vi "Check AI Channel Settings.vi"(8 "error in":errorcluster, 9 "read channel settings":T1[](array[typedef]), 10 "initial channel settings":T1[](array[typedef]), 11 "TestCase in":refnum<class "TestCase.lvclass">) -> (0 "error out":errorcluster, 3 "TestCase out":refnum<class "TestCase.lvclass">)   [LabVIEW 2017, in "Module Test.lvclass"]
uses:
  Module Test Classes/Module Test.lvclass
  Scripting/Modules/Mode Classes/Controls/analog channel settings.ctl
  <vilib>/addons/_JKI Toolkits/VI Tester/TestCase.llb/TestCase.lvclass
  Scripting/Scan Engine Scripting.lvlib
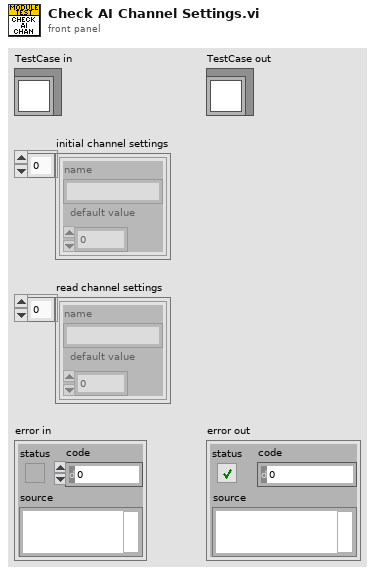
[diagram p1: front panel]
types:
  T1 = typedef "Scan Engine Scripting.lvlib/analog channel settings.ctl" = cluster{"name":string, "default value":dbl}
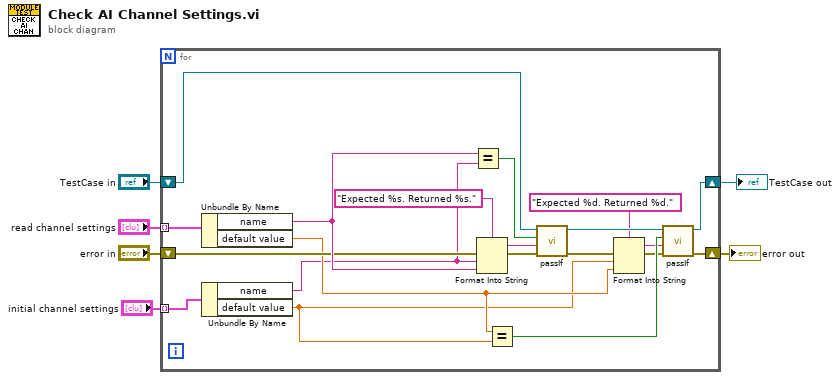
[diagram p0: block diagram]
diagram:
  n1 = for {
    tunnel: "read channel settings" -> [w25] mode=indexing
    tunnel: "initial channel settings" -> [w26] mode=indexing
    shift-right: [w17] -> w3
    shift-left: "TestCase in" -> [w24]
    shift-right: [w13] -> w1
    shift-left: "error in" -> [w21]
    n2 = Unbundle By Name(w25) -> ("name"=w22:string, "default value"=w16:dbl)
    n3 = Unbundle By Name(w26) -> ("name"=w8:string, "default value"=w11:dbl)
    n4 = Equal?(x=w22, y=w8) -> (x = y?=w23:bool)
    n5 = Format Into String(format string="Expected %s. Returned %s.", error in=w21, w8, w22) -> (resulting string=w10:string, error out=w20:errorcluster)  [unwired: 1 in]
    n6 = Equal?(x=w16, y=w11) -> (x = y?=w18:bool)
    n7 = call-dynamic "passIf.vi"("error in (no error)"=w20, "message (\"\")"=w10, "pass"=w23, "TestCase in"=w24) -> ("error out"=w15:errorcluster, "TestCase out"=w19:refnum<class "TestCase.lvclass">)  [unwired: 6 in]
    n8 = Format Into String(format string="Expected %d. Returned %d.", error in=w15, w11, w16) -> (resulting string=w9:string, error out=w14:errorcluster)  [unwired: 1 in]
    n9 = call-dynamic "passIf.vi"("error in (no error)"=w14, "message (\"\")"=w9, "pass"=w18, "TestCase in"=w19) -> ("error out"=w13:errorcluster, "TestCase out"=w17:refnum<class "TestCase.lvclass">)  [unwired: 6 in]
  }
  "TestCase out" <- w3
  "error out" <- w1
